vi "Write Shutdown Microgrid Msg.vi"(10 "Shutdown Microgrid Msg":refnum<class "Shutdown Microgrid Msg.lvclass">, 11 "Remote Operation Abstract in":refnum<class "Remote Operation Abstract.lvclass">) -> (3 "Remote Operation Abstract out":refnum<class "Remote Operation Abstract.lvclass">)   [LabVIEW 2018, in "Remote Operation Abstract.lvlib" / "Remote Operation Abstract.lvclass"]
uses:
  Remote Operation Abstract.lvclass
  Remote Operation Abstract Messages/Shutdown Microgrid Msg/Shutdown Microgrid Msg.lvclass
  Remote Operation Abstract.lvclass/Remote Operation Abstract.ctl
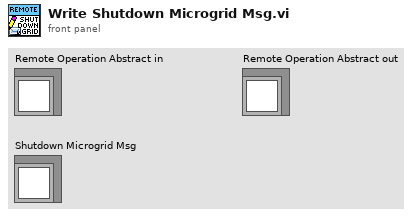
[diagram p1: front panel]
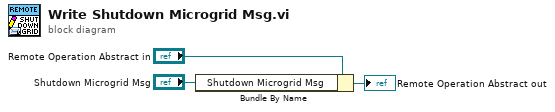
[diagram p0: block diagram]
diagram:
  n1 = Bundle By Name(cluster="Remote Operation Abstract in", "Shutdown Microgrid Msg"="Shutdown Microgrid Msg") -> (→"Remote Operation Abstract out":refnum<class "Remote Operation Abstract.lvclass">)
